vi "QTrkMinimalTest.vi"() -> ()   [LabVIEW 2011]
uses:
  QTrk.llb/QTrkSettings.ctl
  QTrk.llb/QTrkDLL.vi
panel:
  in  "QTrk Settings":T1={"Image width"=150, "Image height"=150, "Number of threads (CPU based)"=-1, "Max Queue Size"=128, "XCOR Profile Length"=32, "XCOR Profile Width"=2, "XCOR Iterations"=5, "ZLUT MinRadius"=50.0, "ZLUT MaxRadius"=64.0, "ZLUT AngularSteps"=0, "QI Iterations"=64, "QI RadialSteps"=64, "QI AngularSteps"=2, "QI MinRadius"=50.0, "QI MaxRadius"=50.0}
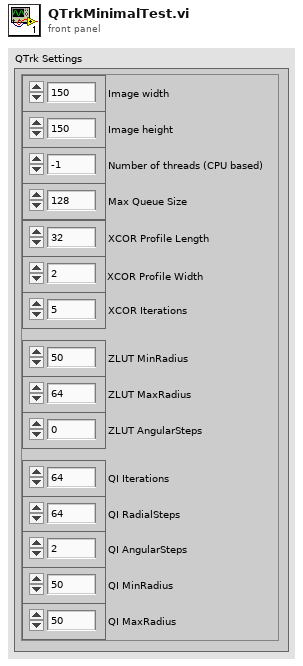
[diagram p1: front panel]
types:
  T1 = typedef "QTrkSettings.ctl" = cluster{"Image width":i32, "Image height":i32, "Number of threads (CPU based)":i32, "Max Queue Size":i32, "XCOR Profile Length":i32, "XCOR Profile Width":i32, "XCOR Iterations":i32, "ZLUT MinRadius":sgl, "ZLUT MaxRadius":sgl, "ZLUT AngularSteps":i32, "QI Iterations":i32, "QI RadialSteps":i32, "QI AngularSteps":i32, "QI MinRadius":sgl, "QI MaxRadius":sgl}
  T2 = typedef "QTrkInstance.ctl" = cluster{"QTrk Pointer":u64, "QTrk Settings":T1}
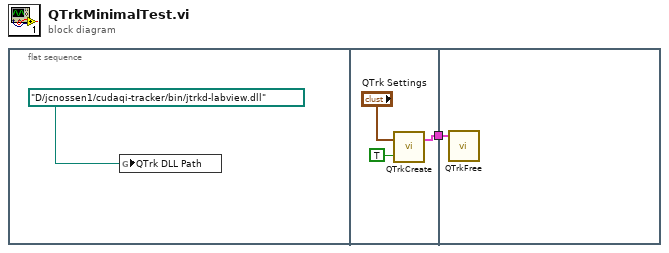
[diagram p0: block diagram]
diagram:
  n1 = flat-sequence {
    tunnel: [w3] -> w1
    tunnel: w1 -> [w6]
    frame #0 {
      n2 = global write "QTrkDLL.vi" "QTrk DLL Path"(path "D:/jcnossen1/cudaqi-tracker/bin/jtrkd-labview.dll") -> ()
    }
    frame #1 {
      n3 = call "QTrkCreate.vi"("startNow"=TRUE, "QTrk Settings"="QTrk Settings") -> ("QTrk Instance"=w3:T2)  [unwired: 1 in]
    }
    frame #2 {
      n4 = call "QTrkFree.vi"("QTrk Instance"=w6) -> ()  [unwired: 5 in]
    }
  }
